vi "Initialize camera.vi"(8 "error in (no error)":errorcluster, 11 "CCD in":refnum<class "CCD.lvclass">) -> (0 "error out":errorcluster, 3 "CCD out":refnum<class "CCD.lvclass">)   [LabVIEW 2018, in "CCD.lvclass"]
uses:
  CCD.lvclass
  CCD.lvclass/CCD.ctl
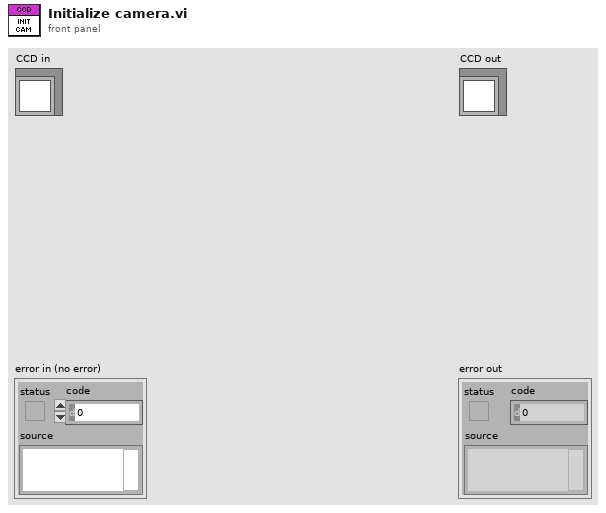
[diagram p1: front panel]
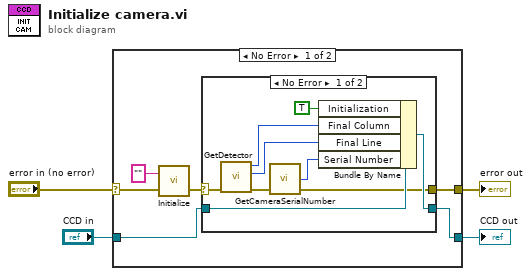
[diagram p0: block diagram]
diagram:
  n1 = case shown="No Error" "error in (no error)" {
    selector: "error in (no error)" -> [w8 w23]
    tunnel: [w5 w23] -> w1
    tunnel: [w6 w22] -> w3
    tunnel: "CCD in" -> [w7 w22]
    frame No Error {
      n2 = call <userlib>:"Initialize.vi"("error in (no error)"=w8, "directory (\"\")"="" ("directory (\"\")")) -> ("error out"=w10:errorcluster)  [unwired: 1 out]
      n3 = case shown="No Error" w10 {
        selector: w10 -> [w14 w21]
        tunnel: w7 -> [w15 w20]
        tunnel: [w13 w20] -> w6
        tunnel: [w12 w21] -> w5
        frame No Error {
          n4 = call <userlib>:"GetDetector.vi"("error in (no error)"=w14) -> ("error out"=w19:errorcluster, "ypixels"=w17:i32, "xpixels"=w16:i32)  [unwired: 3 in, 1 out]
          n5 = call <userlib>:"GetCameraSerialNumber.vi"("error in (no error)"=w19) -> ("error out"=w12:errorcluster, "number"=w18:i32)  [unwired: 2 in, 1 out]
          n6 = Bundle By Name(cluster=w15, "Initialization"=TRUE, "Final Column"=w16, "Final Line"=w17, "Serial Number"=w18) -> (w13:refnum<class "CCD.lvclass">)
        }
        frame Error {
        }
      }
    }
    frame Error {
    }
  }
  "error out" <- w1
  "CCD out" <- w3
